vi "Get Actor Enqueuer.vi"(8 "error in (no error)":errorcluster, 10 "Actor Name":string, 11 "CallActorCenter in":refnum<class "CallActorCenter.lvclass">) -> (0 "error out":errorcluster, 1 "value":refnum<class "Message Enqueuer.lvclass">, 2 "key not found?":bool, 3 "CallActorCenter out":refnum<class "CallActorCenter.lvclass">)   [LabVIEW 2021]
uses:
  CallActorCenter.lvclass
  C:/Program Files (x86)/National Instruments/LabVIEW 2021/user.lib/John_Lib/AbstractActorTemplate/AbstractActorTemplate/UIActorTop.lvclass
  <vilib>/ActorFramework/Message Enqueuer/Message Enqueuer.lvclass
  <userlib>/John_Lib/AbstractActorTemplate/AbstractActorTemplate/UIActorTop.lvclass
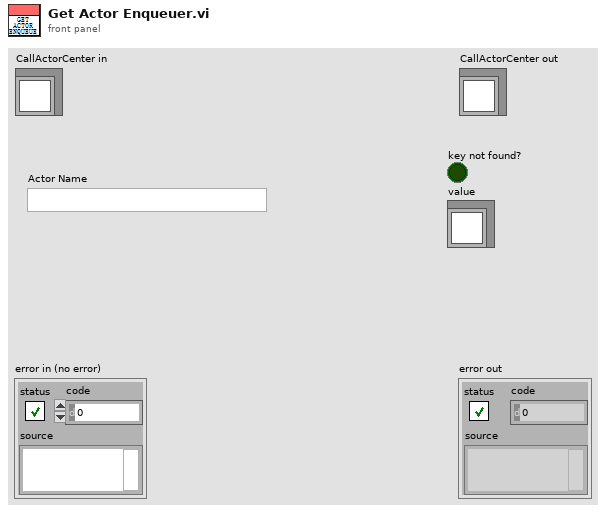
[diagram p1: front panel]
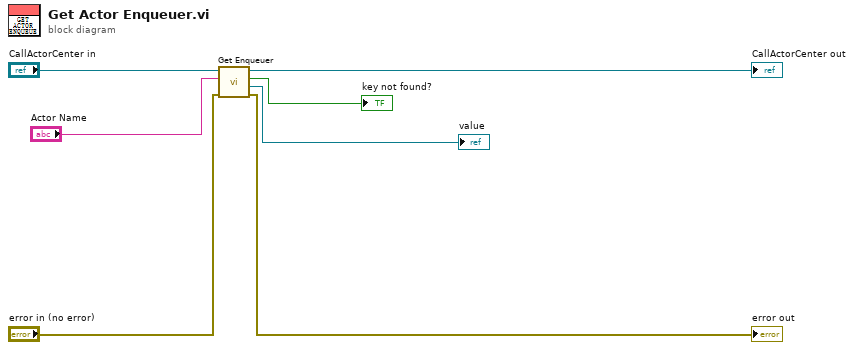
[diagram p0: block diagram]
diagram:
  n1 = call <userlib>:"Get Enqueuer.vi"("error in (no error)"="error in (no error)", "ActorQName"="Actor Name", "UIActorTop in"="CallActorCenter in") -> ("error out"=→"error out":errorcluster, "Nested Actor's Enqueuer"=→"value":refnum<class "Message Enqueuer.lvclass">, "key not found?"=→"key not found?":bool, "UIActorTop out"=→"CallActorCenter out":refnum<class "CallActorCenter.lvclass">)  [unwired: 4 in, 1 out]
